vi "set BK9129B currents x3.vi"(0 "current in 1 (mA)":dbl format="%.2f", 1 "current in 2 (mA)":dbl format="%.2f", 2 "current in 3 (mA)":dbl format="%.2f", 3 "error in":errorcluster, 4 "VISA in":refnum<visa-resource-name>="GPIB0::12::INSTR") -> (5 "VISA out":refnum<visa-resource-name>="GPIB0::12::INSTR", 6 "error out":errorcluster)   [LabVIEW 2019]
panel:
  out "output string":string
  # "inputs"
  # "outputs"
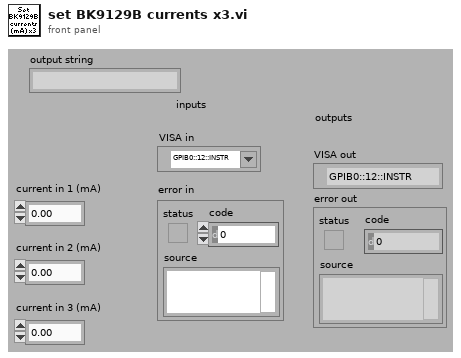
[diagram p1: front panel]
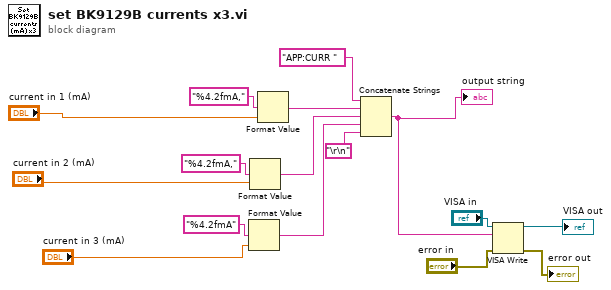
[diagram p0: block diagram]
diagram:
  n1 = Format Value(format string="%4.2fmA" ("string (\"\")"), value (0)="current in 3 (mA)") -> (output string=w13:string)  [unwired: 1 in]
  n2 = Format Value(format string="%4.2fmA," ("string (\"\")"), value (0)="current in 2 (mA)") -> (output string=w12:string)  [unwired: 1 in]
  n3 = Format Value(format string="%4.2fmA," ("string (\"\")"), value (0)="current in 1 (mA)") -> (output string=w11:string)  [unwired: 1 in]
  n4 = Concatenate Strings("APP:CURR " ("format string"), w11, w12, w13, "\r\n") -> (w8:string)
  "output string" <- w8
  n5 = VISA Write(VISA resource name="VISA in", write buffer=w8, error in (no error)="error in") -> (VISA resource name out=→"VISA out":refnum<visa-resource-name>, error out=→"error out":errorcluster)  [unwired: 1 out]
